vi "Write Array of Active Global Channel.vi"(8 "error in (no error)":errorcluster, 10 "Array of Active Global Channel":T1(array[cluster]), 11 "National Instrument USB-6501 in":refnum<class "National Instrument USB-6501.lvclass">) -> (0 "error out":errorcluster, 3 "National Instrument USB-6501 out":refnum<class "National Instrument USB-6501.lvclass">)   [LabVIEW 2016, in "Generic Data Acquisition.lvlib" / "National Instrument USB-6501.lvlib" / "National Instrument USB-6501.lvclass"]
uses:
  National Instrument USB-6501.lvclass
  National Instrument USB-6501.lvclass/National Instrument USB-6501.ctl
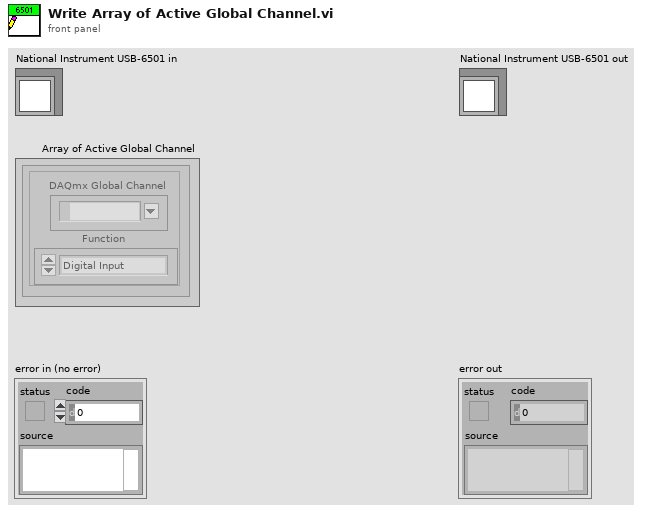
[diagram p1: front panel]
types:
  T1 = cluster{"Function":enum16{"Digital Input", "Digital Output"}, "DAQmx Global Channel":refnum<k21>}[]
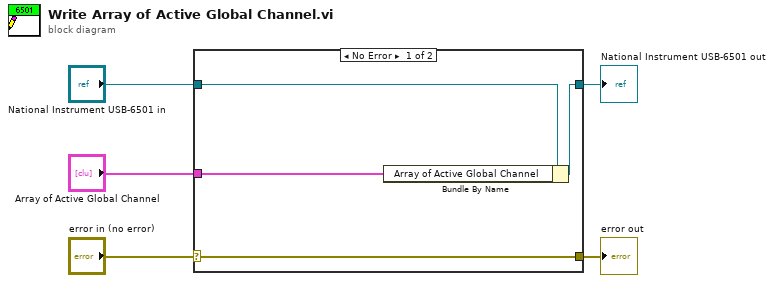
[diagram p0: block diagram]
diagram:
  n1 = case shown="No Error" "error in (no error)" {
    selector: "error in (no error)" -> [w9 w10]
    tunnel: [w9 w10] -> w4
    tunnel: [w7 w11] -> w2
    tunnel: "National Instrument USB-6501 in" -> [w8 w11]
    tunnel: "Array of Active Global Channel" -> [w6 _]
    frame No Error {
      n2 = Bundle By Name(cluster=w8, "Array of Active Global Channel"=w6) -> (w7:refnum<class "National Instrument USB-6501.lvclass">)
    }
    frame Error {
    }
  }
  "error out" <- w4
  "National Instrument USB-6501 out" <- w2
